vi "TagBus_Initialize_Dependency Check.vi"(8 "error in (no error)":errorcluster, 10 "Dependencies Array":T1(array[cluster]), 11 "TagDescriptions in":refnum<class "tag descriptor.lvclass">[](array[class])) -> (0 "error out":errorcluster, 2 "TagDescriptions out":refnum<class "tag descriptor.lvclass">[](array[class]), 3 "Missing Tags":string[](array[string]))   [LabVIEW 2015, in "TagBus.lvclass"]
uses:
  TagBus.lvclass
  <vilib>/NI/Tag Bus/tag/tag descriptor.lvclass
  <vilib>/NI/Tag Bus/tag/tag descriptor.lvclass/tag descriptor.ctl
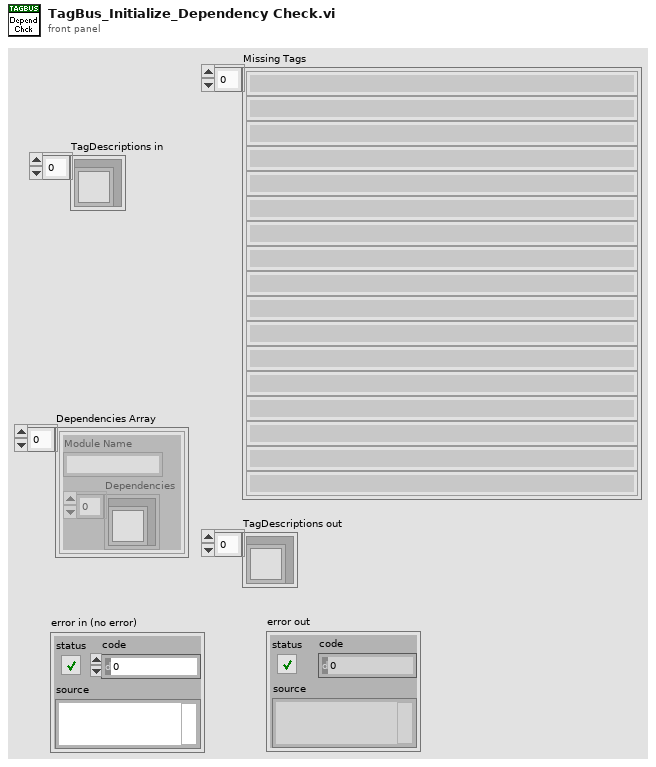
[diagram p1: front panel]
types:
  T1 = cluster{"Module Name":string, "Dependencies":refnum<class "tag descriptor.lvclass">[]}[]
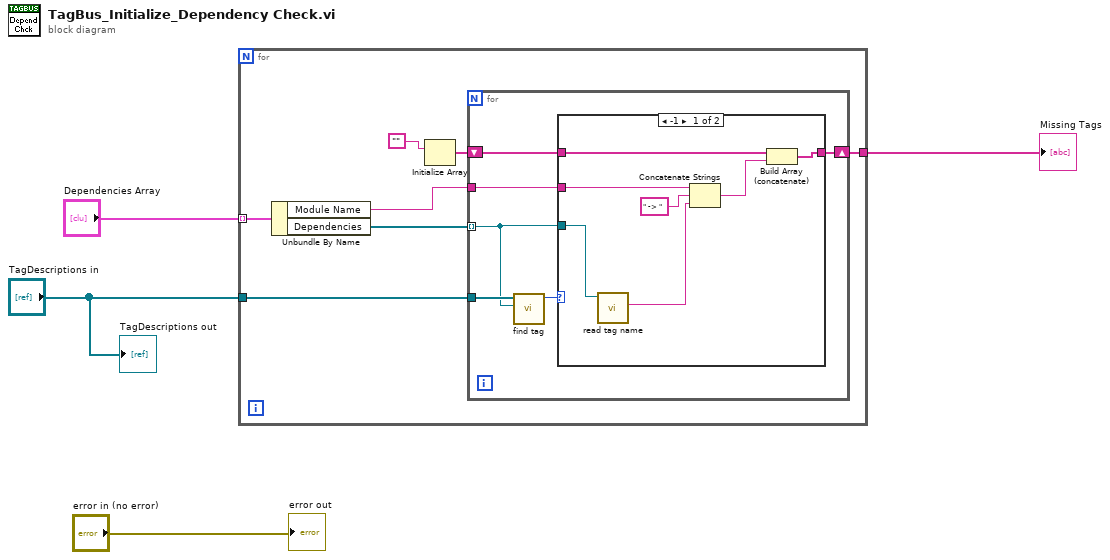
[diagram p0: block diagram]
diagram:
  n1 = for {
    tunnel: [w9] -> w4
    tunnel: "TagDescriptions in" -> [w8]
    tunnel: "Dependencies Array" -> [w7] mode=indexing
    n2 = Unbundle By Name(w7) -> ("Module Name"=w5:string, "Dependencies"=w6:refnum<class "tag descriptor.lvclass">[])
    n3 = Initialize Array("") -> (w11:string[])  [unwired: 1 in]
    n4 = for {
      tunnel: w8 -> [w17]
      tunnel: w6 -> [w16] mode=indexing
      shift-right: [w14] -> w9
      shift-left: w11 -> [w13]
      tunnel: w5 -> [w12]
      n5 = call <vilib>:"find tag.vi"("tag"=w16, "tags in"=w17) -> ("index"=w15:i32)  [unwired: 9 in]
      n6 = case shown="-1" w15 {
        tunnel: w16 -> [w24 _]
        tunnel: [w22 w25] -> w14
        tunnel: w13 -> [w23 w25]
        tunnel: w12 -> [w21 _]
        frame -1 {
          n7 = call <vilib>:"read tag name.vi"("system tag in"=w24) -> ("name"=w20:string)  [unwired: 8 in, 2 out]
          n8 = Concatenate Strings(w21, " -> " ("string"), w20) -> (w19:string)
          n9 = Build Array (concatenate)(w23, w19) -> (w22:string[])
        }
        frame 0, Default {
        }
      }
    }
  }
  "Missing Tags" <- w4
  "error out" <- "error in (no error)"
  "TagDescriptions out" <- "TagDescriptions in"
